vi "Config String to cluster.vi"(8 "error in":errorcluster, 9 "Config":string, 10 "Path":string, 11 "Cluster Ref in":refnum<vi>) -> (3 "Cluster Ref out":refnum<vi>)   [LabVIEW 2012]
uses:
  <vilib>/regexp/Match Regular Expression.xnode
panel:
  out "Config":T1
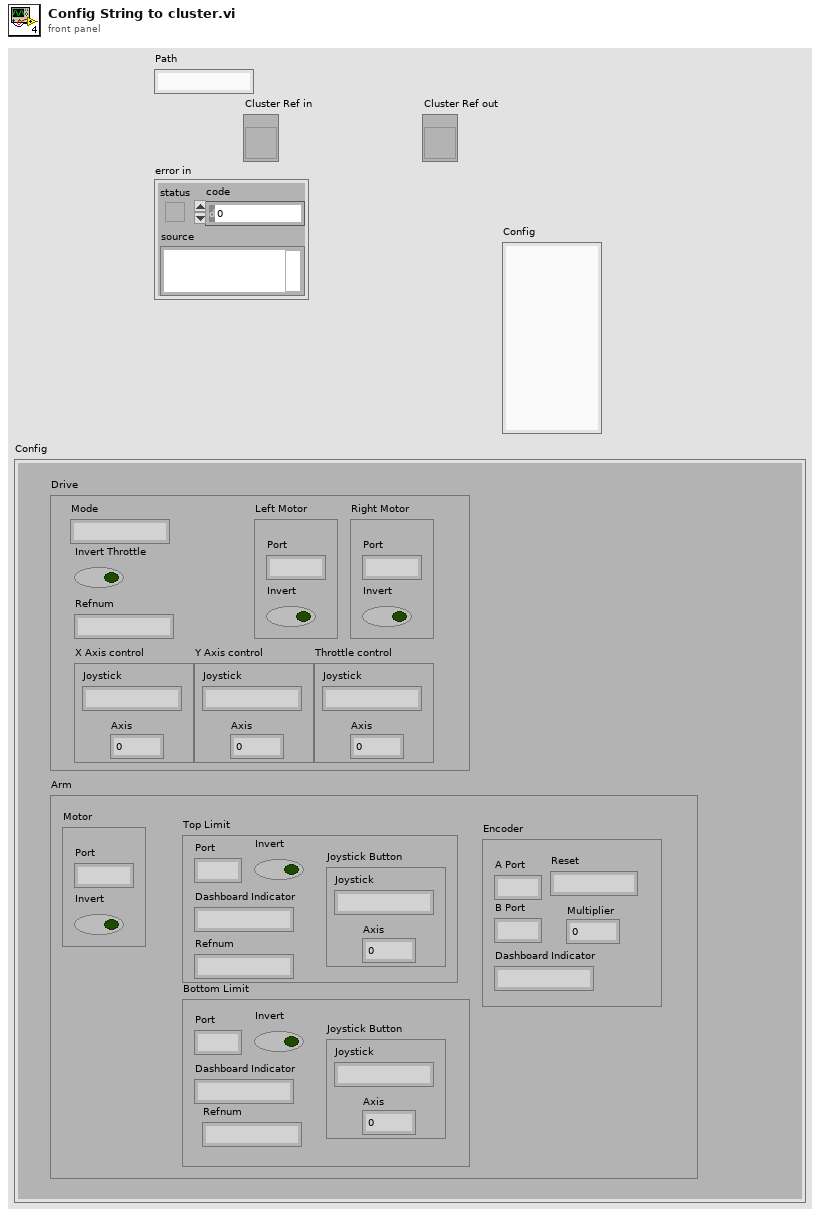
[diagram p1: front panel]
types:
  T1 = cluster{"Drive":cluster{"Mode":string, "Invert Throttle":bool, "Refnum":string, "Left Motor":cluster{"Port":string, "Invert":bool}, "Right Motor":cluster{"Port":string, "Invert":bool}, "X Axis control":cluster{"Joystick":string, "Axis":dbl}, "Y Axis control":cluster{"Joystick":string, "Axis":dbl}, "Throttle control":cluster{"Joystick":string, "Axis":dbl}}, "Arm":cluster{"Motor":cluster{"Port":string, "Invert":bool}, "Top Limit":cluster{"Port":string, "Invert":bool, "Dashboard Indicator":string, "Joystick Button":cluster{"Joystick":string, "Axis":dbl}, "Refnum":string}, "Encoder":cluster{"A Port":string, "B Port":string, "Reset":string, "Multiplier":dbl, "Dashboard Indicator":string}, "Bottom Limit":cluster{"Port":string, "Invert":bool, "Dashboard Indicator":string, "Joystick Button":cluster{"Joystick":string, "Axis":dbl}, "Refnum":string}}}
  T2 = typedef "Type Enum.ctl" = enum8{"Void", "I8", "I16", "I32", "I64", "U8", "U16", "U32", "U64", "Single Float", "Double Float", "Extended Float", "Single Complex", "Double Complex", "Extended Complex", "Enum I8 NEVER", "Enum I16 NEVER", "Enum I32 NEVER", "Enum I64 NEVER", "Enum U8", "Enum U16", "Enum U32", "Enum U64", "Single Float With Unit", "Double Float With Unit", "Extended Float With Unit", "Single Complex With Unit", "Double Complex With Unit", "Extended Complex With Unit", "boolU16", "Boolean", "String", "Handle", "Path", "Picture", "C String", "Pascal String", "Tag", "SubString", "Array", "SubArray", "Cluster", "Numeric Cluster", "Variant", "LV Variant", "Measure Data (waveform)", "Refnum", "ExtData", "function", "Typedef", "Poly VI", "bad wire", "LabVIEW Class Instance"}
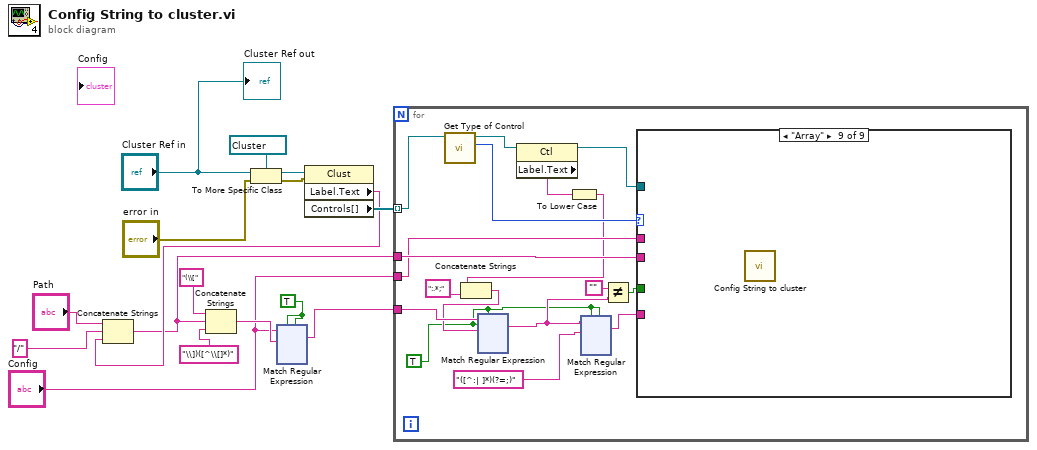
[diagram p0: block diagram]
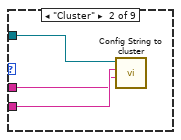
[diagram p3: hidden frame]
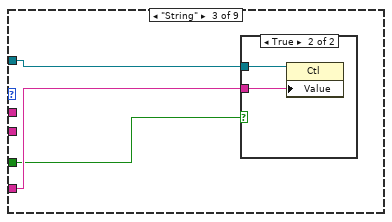
[diagram p4: hidden frame]
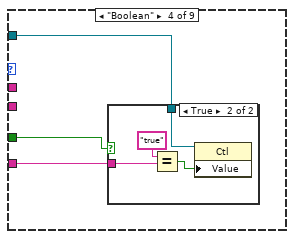
[diagram p6: hidden frame]
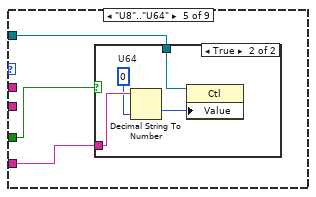
[diagram p8: hidden frame]
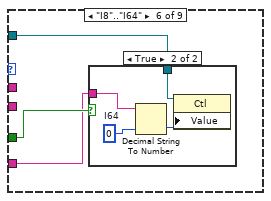
[diagram p10: hidden frame]
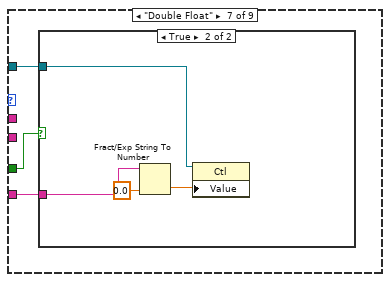
[diagram p12: hidden frame]
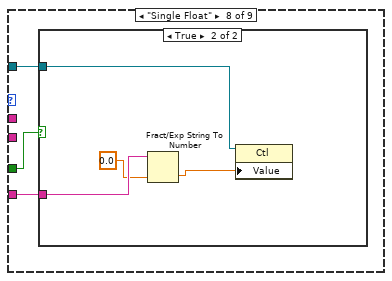
[diagram p14: hidden frame]
diagram:
  w1 = TRUE
  n1 = To More Specific Class(target class=refnum<vi> refnum ("reference"), reference="Cluster Ref in", error in="error in") -> (specific class reference=w15:refnum<vi>, error out=w14:errorcluster)
  n2 = property class="Clust"(reference=w15, error in=w14) -> ("Label.Text"=w8:string, "Controls[]"=w12:refnum<vi>[])  [unwired: 2 out]
  n3 = Concatenate Strings("Path", "/", w8) -> (w5:string)
  n4 = Concatenate Strings("(\\[", w5, "\\])([^\\[]*)") -> (w11:string)
  n5 = xnode "Match Regular Expression"("input string"="Config", "regular expression"=w11, "ignore case? (F)"=w1, "multiline? (F)"=w1) -> ("whole match"=w3:string)  [unwired: 2 in, 4 out]
  n6 = for {
    tunnel: w12 -> [w33] mode=indexing
    tunnel: w5 -> [w30]
    tunnel: "Config" -> [w28]
    tunnel: w3 -> [w22]
    w17 = TRUE
    n7 = call <vilib>:"Get Type of Control.vi"("Control Ref In"=w33) -> ("Type Enum"=w32:T2, "Control Ref Out"=w31:refnum<vi>)  [unwired: 8 in, 1 out]
    n8 = property class="Ctl"(reference=w31) -> (reference out=w29:refnum<vi>, "Label.Text"=w27:string)  [unwired: 1 in, 1 out]
    n9 = To Lower Case(string=w27) -> (all lower case string=w26:string)
    n10 = Concatenate Strings(w26, ":.*;") -> (w21:string)
    n11 = xnode "Match Regular Expression"("input string"=w22, "regular expression"=w21, "ignore case? (F)"=w17, "multiline? (F)"=w17) -> ("whole match"=w18:string)  [unwired: 2 in, 4 out]
    n12 = xnode "Match Regular Expression"("input string"=w18, "regular expression"="([^:| ]*)(?=;)", "ignore case? (F)"=w17, "multiline? (F)"=w17) -> ("whole match"=w20:string)  [unwired: 2 in, 4 out]
    n13 = Not Equal?(x="", y=w18) -> (x != y?=w23:bool)
    n14 = case shown="\"Array\"" w32 {
      tunnel: w29 -> [_ w258 w261 w264 w271 w278 w285 w292 _]
      tunnel: w30 -> [_ w257 _ _ _ _ _ _ _]
      tunnel: w28 -> [_ w256 _ _ _ _ _ _ _]
      tunnel: w20 -> [_ _ w260 w266 w272 w279 w286 w293 _]
      tunnel: w23 -> [_ _ w259 w265 w273 w280 w287 w294 _]
      frame "Void", Default {
      }
      frame "Cluster" {
        n15 = call "Config String to cluster.vi"("Config"=w256, "Path"=w257, "Cluster Ref in"=w258) -> ()  [unwired: 8 in, 1 out]
      }
      frame "String" {
        n16 = case shown="True" w259 {
          tunnel: w261 -> [_ w263]
          tunnel: w260 -> [_ w262]
          frame False {
          }
          frame True {
            n17 = property class="Ctl"(reference=w263, "Value"=w262) -> ()  [unwired: 1 in, 2 out]
          }
        }
      }
      frame "Boolean" {
        n18 = case shown="True" w265 {
          tunnel: w266 -> [_ w270]
          tunnel: w264 -> [_ w267]
          frame False {
          }
          frame True {
            n19 = Equal?(x="true", y=w270) -> (x = y?=w268:bool)
            n20 = property class="Ctl"(reference=w267, "Value"=w268) -> ()  [unwired: 1 in, 2 out]
          }
        }
      }
      frame "U8".."U64" {
        n21 = case shown="True" w273 {
          tunnel: w272 -> [_ w277]
          tunnel: w271 -> [_ w275]
          frame False {
          }
          frame True {
            w276 = u64 0  # U64
            n22 = Decimal String To Number(string=w277, default (0L)=w276) -> (number=w274:u64)  [unwired: 1 in, 1 out]
            n23 = property class="Ctl"(reference=w275, "Value"=w274) -> ()  [unwired: 1 in, 2 out]
          }
        }
      }
      frame "I8".."I64" {
        n24 = case shown="True" w280 {
          tunnel: w279 -> [_ w284]
          tunnel: w278 -> [_ w282]
          frame False {
          }
          frame True {
            w283 = i64 0  # I64
            n25 = Decimal String To Number(string=w284, default (0L)=w283) -> (number=w281:i64)  [unwired: 1 in, 1 out]
            n26 = property class="Ctl"(reference=w282, "Value"=w281) -> ()  [unwired: 1 in, 2 out]
          }
        }
      }
      frame "Double Float" {
        n27 = case shown="True" w287 {
          tunnel: w286 -> [_ w291]
          tunnel: w285 -> [_ w288]
          frame False {
          }
          frame True {
            n28 = Fract/Exp String To Number(string=w291, default (0 dbl)=0.0) -> (number=w289:dbl)  [unwired: 2 in, 1 out]
            n29 = property class="Ctl"(reference=w288, "Value"=w289) -> ()  [unwired: 1 in, 2 out]
          }
        }
      }
      frame "Single Float" {
        n30 = case shown="True" w294 {
          tunnel: w293 -> [_ w298]
          tunnel: w292 -> [_ w295]
          frame False {
          }
          frame True {
            n31 = Fract/Exp String To Number(string=w298, default (0 dbl)=sgl 0.0) -> (number=w296:sgl)  [unwired: 2 in, 1 out]
            n32 = property class="Ctl"(reference=w295, "Value"=w296) -> ()  [unwired: 1 in, 2 out]
          }
        }
      }
      frame "Array" {
        n33 = call "Config String to cluster.vi"() -> ()  [unwired: 11 in, 1 out]
      }
    }
  }
  "Cluster Ref out" <- "Cluster Ref in"
